vi "Check Error.vi"(6 "Error on Zero? (f)":bool=TRUE, 7 "Description":string, 10 "Return Code":u32, 11 "error in (no error)":errorcluster) -> (3 "error out":errorcluster)   [LabVIEW 2025, in "Test Unit.lvlib"]
uses:
  Test Unit.lvlib
  <vilib>/Utility/error.llb/Error Cluster From Error Code.vi
  <vilib>/ErrorRing/Error Ring.xnode
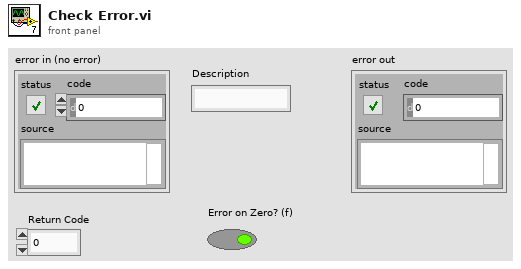
[diagram p1: front panel]
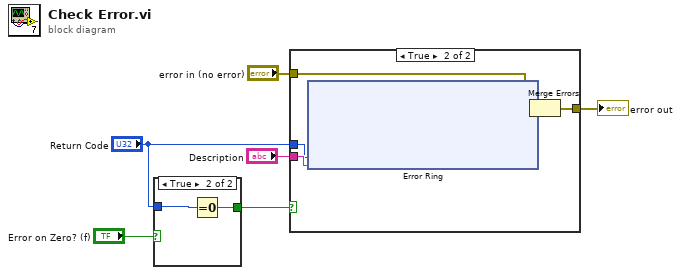
[diagram p0: block diagram]
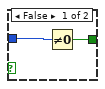
[diagram p2: hidden frame]
diagram:
  n1 = case shown="True" "Error on Zero? (f)" {
    tunnel: "Return Code" -> [w8 w10]
    tunnel: [w7 w9] -> w2
    frame False {
      n2 = Not Equal To 0?(x=w8) -> (x != 0?=w7:bool)
    }
    frame True {
      n3 = Equal To 0?(x=w10) -> (x = 0?=w9:bool)
    }
  }
  n4 = case shown="True" w2 {
    tunnel: "Description" -> [_ w16]
    tunnel: "error in (no error)" -> [w11 w15]
    tunnel: [w11 w14] -> w4
    tunnel: "Return Code" -> [_ w12]
    frame False {
    }
    frame True {
      n5 = xnode "Error Ring"("parameter 0"=w12, "parameter 1"=w16) -> ("error out"=w13:errorcluster)
      n6 = Merge Errors(w15, w13) -> (w14:errorcluster)
    }
  }
  "error out" <- w4
